vi "TT_Width.vi"(7 "Calibrated Image in":T10(plugin-control), 8 "error in (no error)":errorcluster, 10 "TT side Width Input Cluster":T9 {"Reference ROI Before Transformation"."Contours"."Type" items=["No Selection", "Point", "Line", "Rectangle", "Oval", "Polygon", "Freehand Region", "Annulus", "Unused2", "Unused3", "Broken Line", "Freehand Line", "Rotated Rectangle"]; "Measurement ROI-1 Before transformation"."Contours"."Type" items=["No Selection", "Point", "Line", "Rectangle", "Oval", "Polygon", "Freehand Region", "Annulus", "Unused2", "Unused3", "Broken Line", "Freehand Line", "Rotated Rectangle"]; "Ref Line Edge Options"."Edge Polarity" items=["All Edges", "Rising Edges", "Falling Edges"]; "Ref Line Edge Options"."Minimum Edge Strength" format="%.2f"; "Ref Line Edge Options"."Width" step=2; "Ref Line Edge Options"."Kernel Size" step=2; "Ref Line Options"."Min. Points (%)" min=0.0 max=100.0; "Ref Line Options"."Min. SNR (db)" min=0.0; "Ref Line Options"."Max. Score" min=0.0 max=1024.0; "Ref Line Options"."Min. Score" min=0.0 max=1024.0 step=1.0; "Meas ROI-1 Edge Options"."Edge Polarity" items=["All Edges", "Rising Edges", "Falling Edges"]; "Meas ROI-1 Edge Options"."Minimum Edge Strength" format="%.2f"; "Meas ROI-1 Edge Options"."Width" step=2; "Meas ROI-1 Edge Options"."Kernel Size" step=2}, 11 "Image In":T10) -> (0 "error out":errorcluster, 1 "Measurement 1":sgl, 3 "Angle (Pixel)":dbl, 4 "Array points for Arrow overlay":cluster{"X":sgl, "Y":sgl}[](array[cluster]), 5 "Overlay Arrow Lines":T1)   [LabVIEW 2019, in "Algorithm.lvclass"]
uses:
  FrameworkOverrides/Algorithm.lvclass
  <vilib>/vision/NI_Vision_Development_Module.lvlib
  <vilib>/vision/Measure.llb/Edge Polarity.ctl
  <vilib>/vision/Measure.llb/Edge Options.ctl
  <vilib>/vision/Image Controls.llb/IMAQ Image.ctl
  <vilib>/vision/Measure.llb/Straight Edge Process.ctl
  <vilib>/vision/Measure.llb/Straight Edge Options.ctl
panel:
  out "Second Overlay Line":T2
  out "First Overlay Line":T3
  # "INPUT"
  # "OUTPUT"
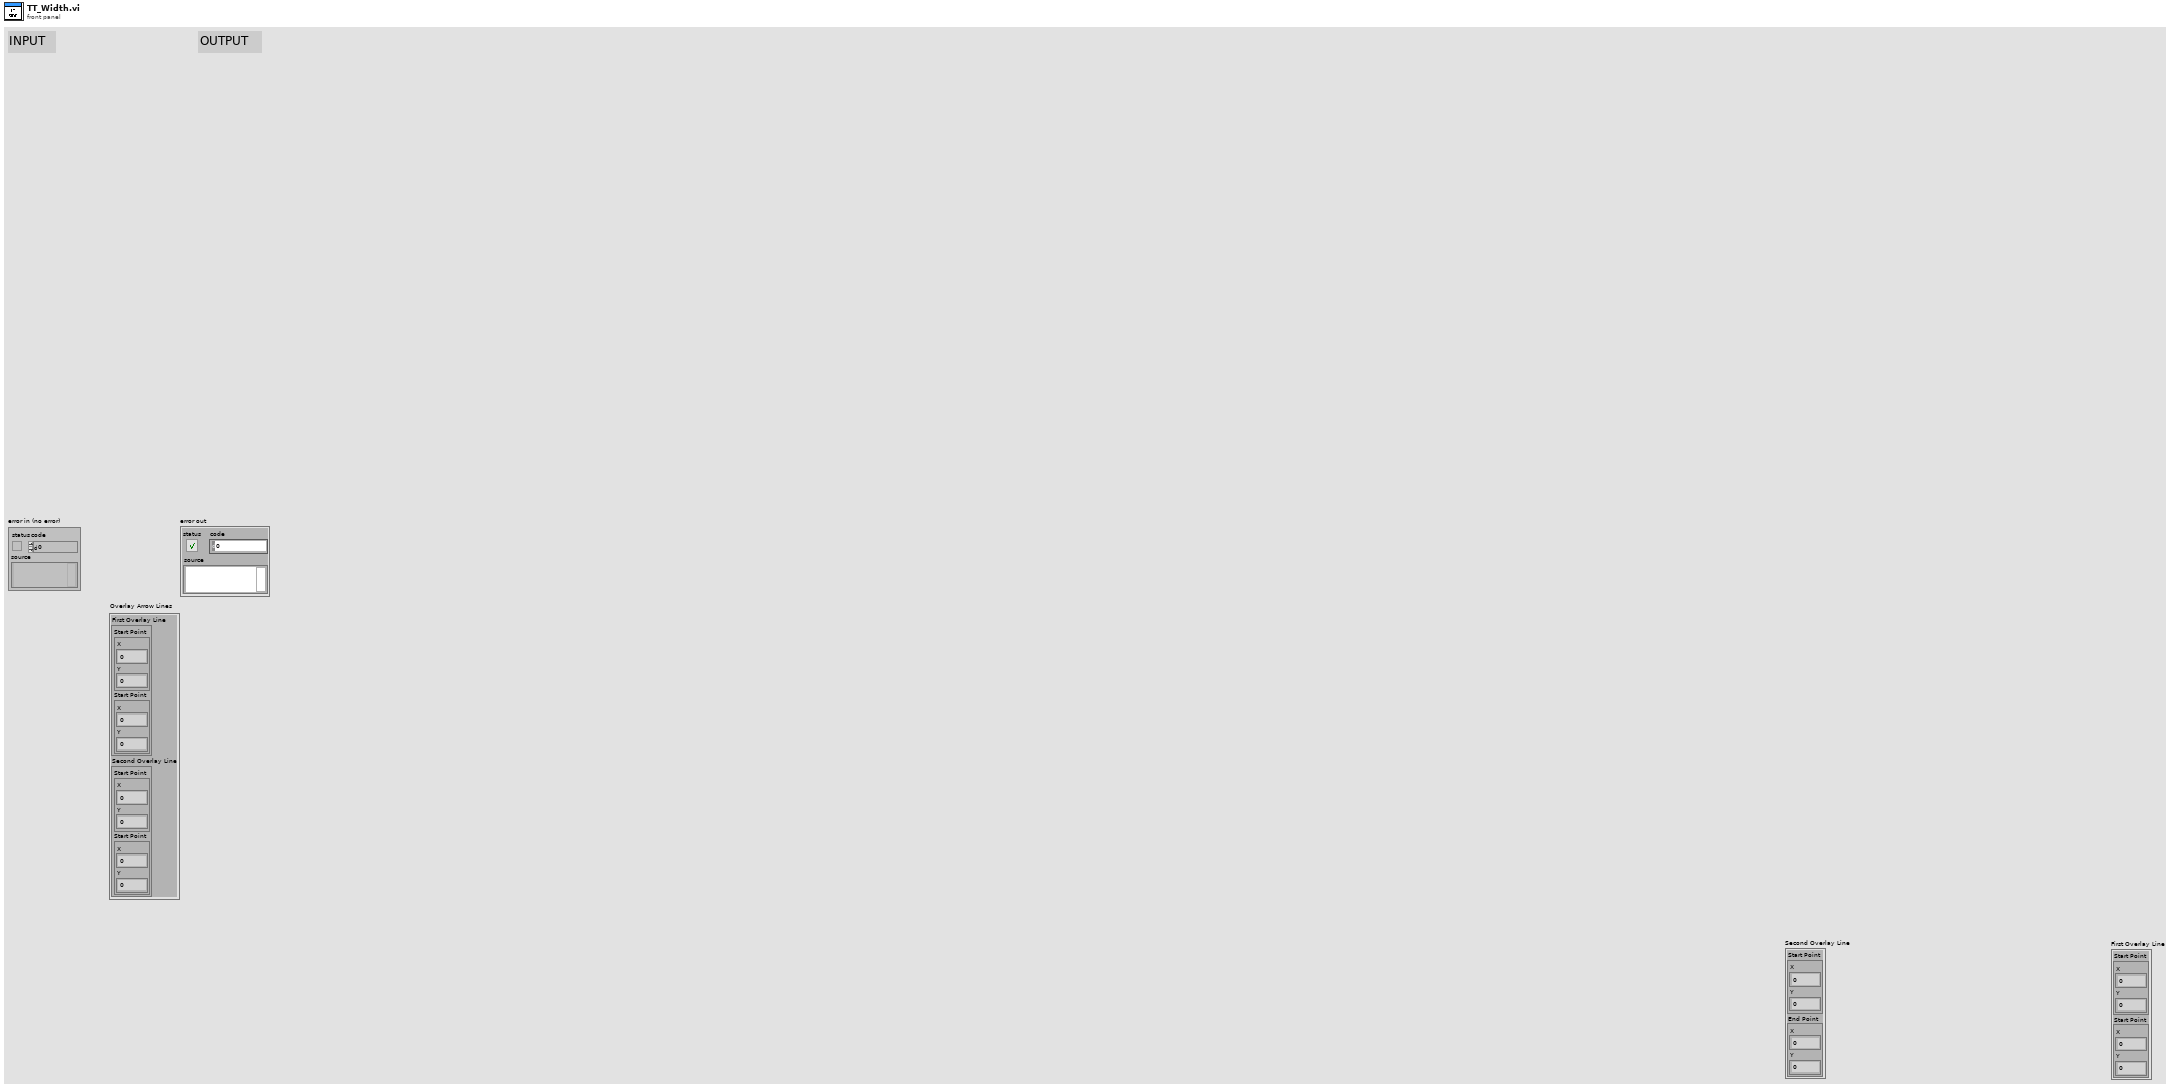
[diagram p1: front panel]
types:
  T1 = cluster{"First Overlay Line ":cluster{"Start Point":cluster{"X":sgl, "Y":sgl}, "Start Point":cluster{"X":sgl, "Y":sgl}}, "Second Overlay Line ":cluster{"Start Point":cluster{"X":sgl, "Y":sgl}, "Start Point":cluster{"X":sgl, "Y":sgl}}}
  T2 = cluster{"Start Point":cluster{"X":sgl, "Y":sgl}, "End Point":cluster{"X":sgl, "Y":sgl}}
  T3 = cluster{"Start Point":cluster{"X":sgl, "Y":sgl}, "Start Point":cluster{"X":sgl, "Y":sgl}}
  T4 = typedef "ROI Descriptor" = cluster{"Global Rectangle":i32[], "Contours":cluster{"ID":enum32{"External", "Internal"}, "Type":u32, "Coordinates":i32[]}[]}
  T5 = typedef "Edge Options.ctl" = cluster{"Edge Polarity":T6, "Kernel Size":u32, "Width":u32, "Minimum Edge Strength":sgl, "Interpolation Type":enum32{"Zero Order", "Bilinear", "Quadratic", "Cubic", "Bilinear Fixed"}, "Data Processing Method":enum32{"Average", "Median"}}
  T6 = typedef "Edge Polarity.ctl" = u32
  T7 = typedef "Straight Edge Options.ctl" = cluster{"Number of Lines":i32, "Type":T8, "Min. Score":dbl, "Max. Score":dbl, "Orientation":dbl, "Angle Range":dbl, "Angle Tolerance":dbl, "Step Size":u32, "Min. SNR (db)":dbl, "Min. Points (%)":dbl, "Hough Iterations":i32}
  T8 = typedef "Straight Edge Process.ctl" = enum32{"First Edge Rake", "Best Edge Rake", "Hough Edge Rake", "First Edge Projection", "Best Edge Projection"}
  T9 = cluster{"AvgMinMax":enum16{"Average", "Max", "Min", "Max2"}, "Center X &Y":cluster{"Center X":dbl, "Center Y":dbl}, "Reference ROI Before Transformation":T4, "Measurement ROI-1 Before transformation":T4, "Ref Line Edge Options":T5, "Ref Line Search Direction":u32, "Ref Line Options":T7, "Meas ROI-1 Edge Options":T5, "Meas ROI-1 Step Size":u32, "Meas ROI-1 Scan Direction":u16, "Meas ROI-1 Process":enum16{"Get First Edge", "Get First + Last Edge", "Get All Edges", "Get Best Edge"}, "OverlayOptions":cluster{"OverlayEnable":bool, "OverlayText":string, "OverlayCoords":i32[], "OverlayAngle":i32, "OverlayTextSize":i32, "OverlayTextColor":string, "OverlayROI":bool, "OverlayRakeLine":bool, "OverlayPoints":bool}}
  T10 = typedef "IMAQ Image.ctl" = refnum<image>
  T11 = cluster{"Left":dbl, "Top":dbl, "Right":dbl, "Bottom":dbl, "Angle":dbl}
  T12 = cluster{"Search Direction":u32, "Edge Options":T5, "Show Search Area":bool, "Show Search Lines":bool, "Show Edges Found":bool, "Show Result":bool, "Search Area Color":u32, "Search Lines Color":u32, "Edge Locations Color":u32, "Result Color":u32, "Overlay Group Name":string}
  T13 = enum16{"Get First Edge", "Get First + Last Edge", "Get All Edges", "Get Best Edge"}
  T14 = cluster{"OverlayEnable":bool, "OverlayText":string, "OverlayCoords":i32[], "OverlayAngle":i32, "OverlayTextSize":i32, "OverlayTextColor":string, "OverlayROI":bool, "OverlayRakeLine":bool, "OverlayPoints":bool}
  T15 = cluster{"ID":enum32{"External", "Internal"}, "Type":u32, "Coordinates":i32[]}[]
  T16 = cluster{"ID":enum32{"External", "Internal"}, "Type":u32, "Coordinates":i32[]}
  T17 = cluster{"Coordinates[0]":i32, "Coordinates[1]":i32, "Coordinates[2]":i32, "Coordinates[3]":i32, "Coordinates[4]":i32}
  T18 = cluster{"Point1 (Pixels)":cluster{"X":sgl, "Y":sgl}, "Point2 (Pixels)":cluster{"X":sgl, "Y":sgl}, "Point1 (Real-World)":cluster{"X":sgl, "Y":sgl}, "Point2 (Real-World)":cluster{"X":sgl, "Y":sgl}, "Angle (Pixel)":dbl, "Angle (Real-World)":dbl, "Score":dbl, "Straightness":dbl, "Average SNR (db)":dbl, "Calibration Valid":bool}[]
  T19 = cluster{"Point1 (Pixels)":cluster{"X":sgl, "Y":sgl}, "Point2 (Pixels)":cluster{"X":sgl, "Y":sgl}, "Point1 (Real-World)":cluster{"X":sgl, "Y":sgl}, "Point2 (Real-World)":cluster{"X":sgl, "Y":sgl}, "Angle (Pixel)":dbl, "Angle (Real-World)":dbl, "Score":dbl, "Straightness":dbl, "Average SNR (db)":dbl, "Calibration Valid":bool}
  T20 = typedef "Edge New.ctl" = cluster{"Location (Pixel)":cluster{"X":sgl, "Y":sgl}, "Location (Real-World)":cluster{"X":sgl, "Y":sgl}, "Distance (Pixel)":dbl, "Distance (Real-World)":dbl, "Strength":dbl, "Noise":dbl, "Rising?":bool}
  T21 = typedef "Search Line.ctl" = cluster{"Start Point":cluster{"X":sgl, "Y":sgl}, "End Point":cluster{"X":sgl, "Y":sgl}, "Edge Info":T20[], "Edge Map":dbl[], "Calibration Valid":bool}
  T22 = cluster{"Start Point":cluster{"X":sgl, "Y":sgl}, "Location (Pixel)":cluster{"X":sgl, "Y":sgl}}
  T23 = cluster{"Location (Pixel)":cluster{"X":sgl, "Y":sgl}, "End Point":cluster{"X":sgl, "Y":sgl}}
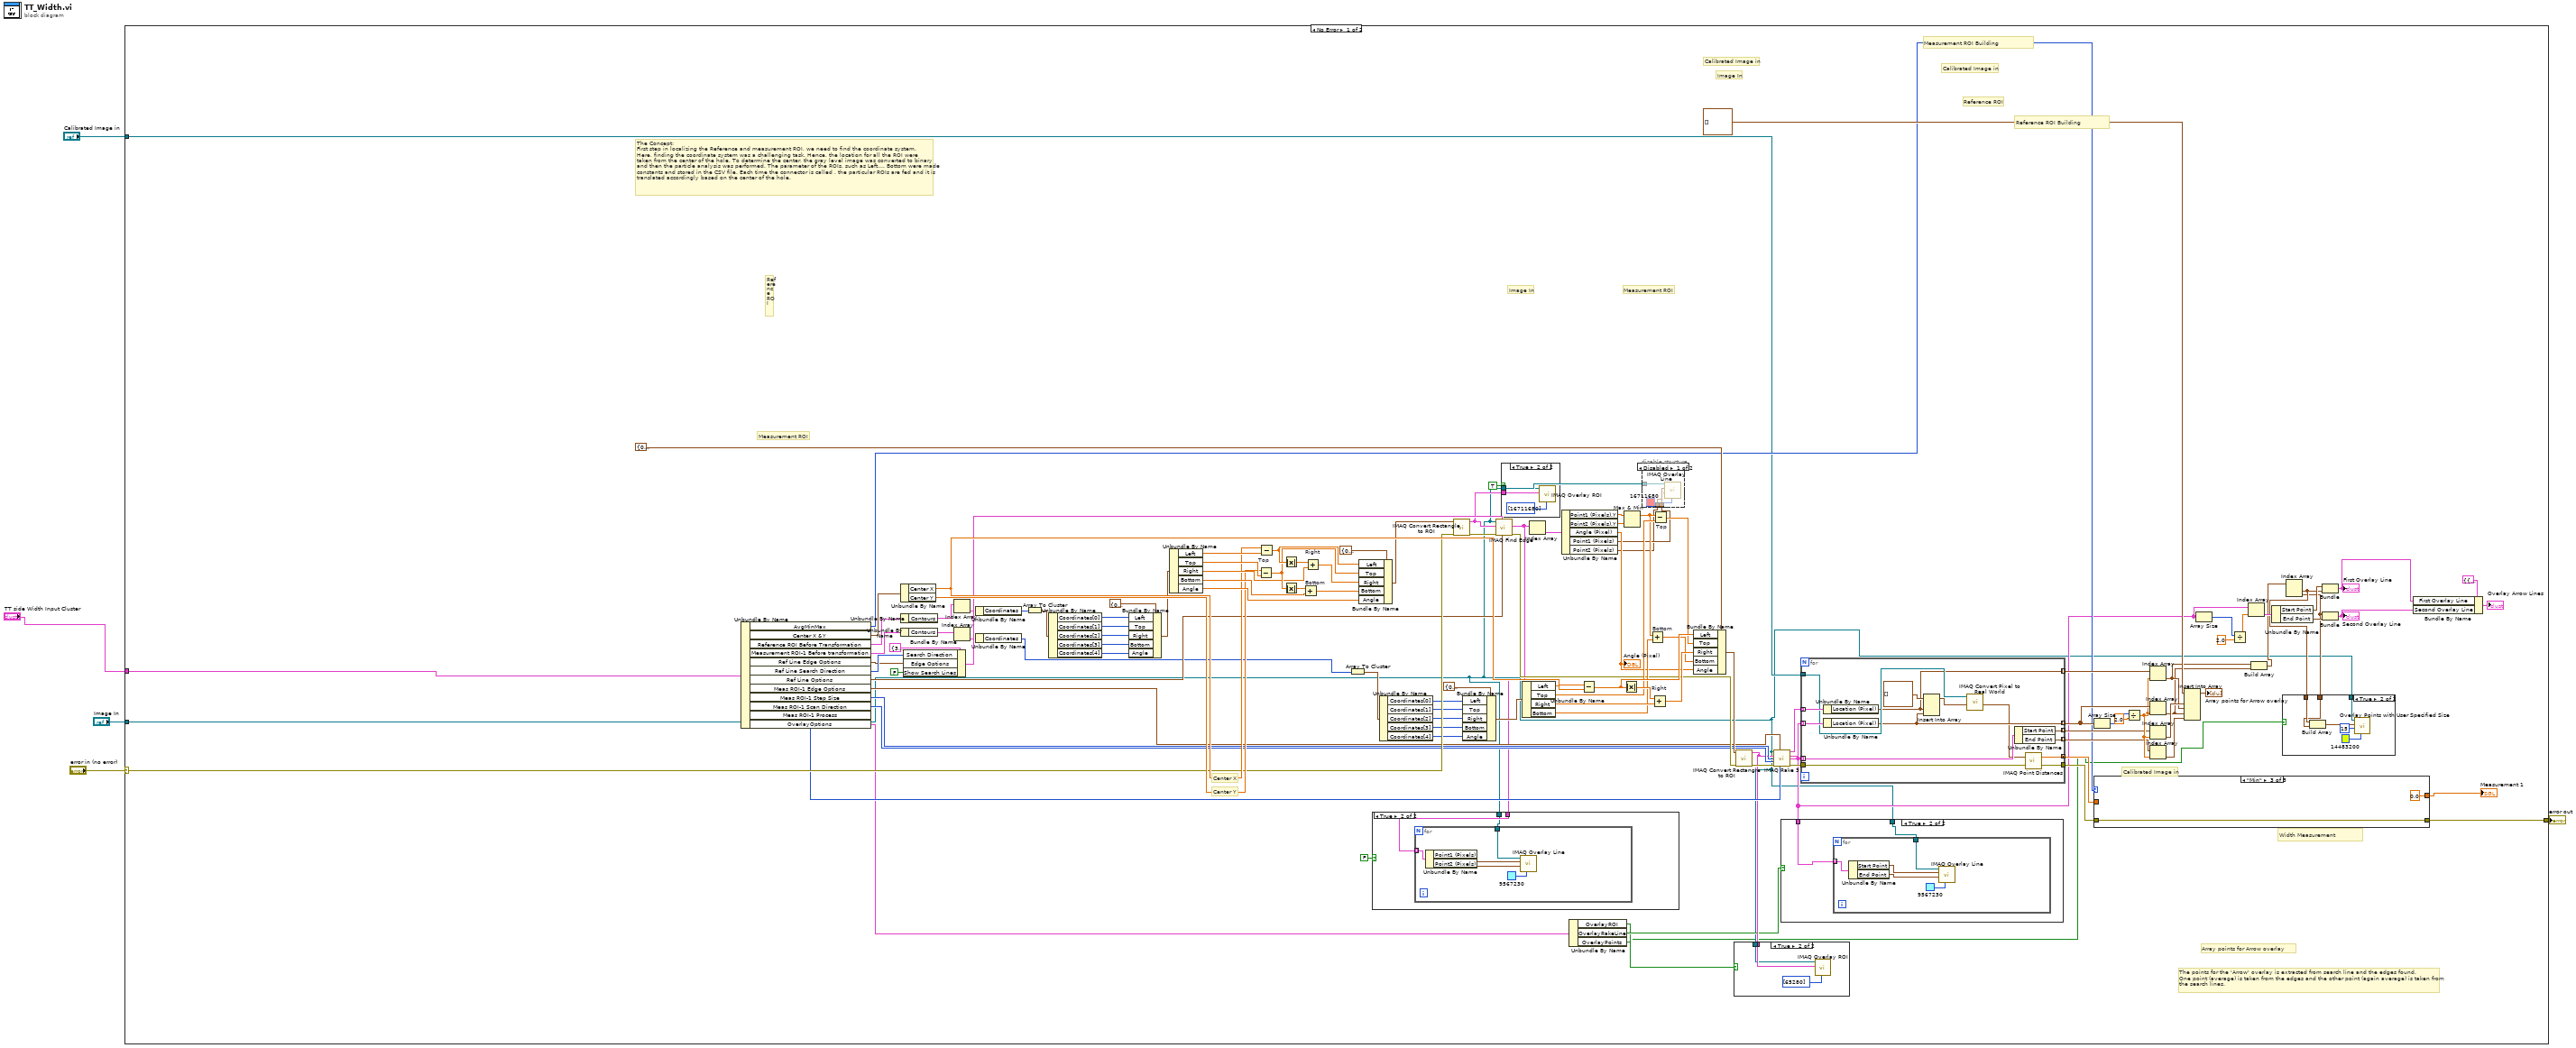
[diagram p0: block diagram]
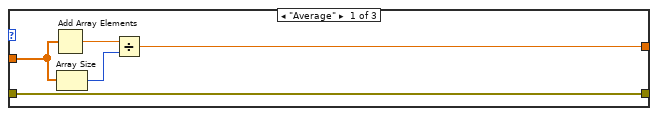
[diagram p8: hidden frame]
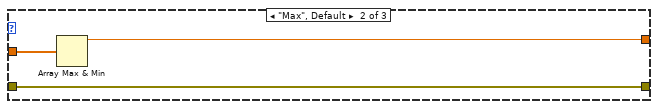
[diagram p9: hidden frame]
diagram:
  n1 = case shown="No Error" "error in (no error)" {
    selector: "error in (no error)" -> [w79 w179]
    tunnel: "Image In" -> [w9 _]
    tunnel: [w91 w179] -> w4
    tunnel: "Calibrated Image in" -> [w37 _]
    tunnel: "TT side Width Input Cluster" -> [w72 _]
    frame No Error {
      # "The points for the 'Arrow' overlay is extracted from search line and the edges found.\nOne point (average) is taken from the edges and the other point (again average) is taken from \nthe search lines."
      # "Array points for Arrow overlay"
      # "The Concept:\nFirst step in localizing the Reference and measurement ROI, we need to find the coordinate system.\nHere, finding the coordinate system was a challenging task. Hence, the location for all the ROI were \ntaken from the center of the hole. To determine the center, the gray level image was converted to binary\nand then the particle analysis was performed. The parameter of the ROIs, such as Left.... Bottom were made \nconstants and stored in the CSV file. Each time the connector is called , the particular ROIs are fed and it is\ntranslated accordingly based on the center of the hole."
      # "Calibrated Image in"
      # "Image In"
      # "Calibrated Image in"
      # "Image In"
      # "Calibrated Image in"
      # "Center Y"
      # "Center X"
      # "Reference ROI"
      # "Measurement ROI"
      # "Width Measurement"
      # "Reference ROI"
      # "Measurement ROI"
      # "Measurement ROI Building"
      # "Reference ROI Building"
      n2 = Unbundle By Name(w72) -> ("AvgMinMax"=w63:enum16{"Average", "Max", "Min", "Max2"}, "Center X &Y"=w62:cluster{"Center X":dbl, "Center Y":dbl}, "Reference ROI Before Transformation"=w56:T4, "Measurement ROI-1 Before transformation"=w46:T4, "Ref Line Edge Options"=w70:T5, "Ref Line Search Direction"=w71:u32, "Ref Line Options"=w68:T7, "Meas ROI-1 Edge Options"=w67:T5, "Meas ROI-1 Step Size"=w66:u32, "Meas ROI-1 Scan Direction"=w65:u16, "Meas ROI-1 Process"=w64:T13, "OverlayOptions"=w28:T14)
      n3 = Unbundle By Name(w62) -> ("Center X"=w81:dbl, "Center Y"=w80:dbl)
      n4 = Unbundle By Name(w56) -> ("Contours"=w55:T15)
      n5 = Unbundle By Name(w46) -> ("Contours"=w59:T15)
      n6 = Bundle By Name(cluster=T12 {"Search Direction"=3, "Edge Options"={"Edge Polarity"=0, "Kernel Size"=3, "Width"=3, "Minimum Edge Strength"=50.0, "Interpolation Type"=enum."Zero Order", "Data Processing Method"=enum."Average"}, "Show Search Area"=FALSE, "Show Search Lines"=FALSE, "Show Edges Found"=FALSE, "Show Result"=FALSE, "Search Area Color"=65280, "Search Lines Color"=255, "Edge Locations Color"=16776960, "Result Color"=16711680, "Overlay Group Name"=""} ("Options"), "Search Direction"=w71, "Edge Options"=w70, "Show Search Lines"=FALSE) -> (w69:T12)
      n7 = Index Array(array=w55) -> (element=w57:T16)  [unwired: 1 in]
      n8 = Index Array(array=w59) -> (element=w60:T16)  [unwired: 1 in]
      n9 = Unbundle By Name(w57) -> ("Coordinates"=w58:i32[])
      n10 = Unbundle By Name(w60) -> ("Coordinates"=w61:i32[])
      n11 = Array To Cluster(array=w58) -> (cluster=w53:T17)
      n12 = Unbundle By Name "Unbundle By Name"(w53) -> ("Coordinates[0]"=w52:i32, "Coordinates[1]"=w51:i32, "Coordinates[2]"=w50:i32, "Coordinates[3]"=w49:i32, "Coordinates[4]"=w48:i32)
      n13 = Bundle By Name(cluster=T11 {"Left"=0.0, "Top"=0.0, "Right"=0.0, "Bottom"=0.0, "Angle"=0.0} ("Measurement ROI-1 Before transformation"), "Left"=w52, "Top"=w51, "Right"=w50, "Bottom"=w49, "Angle"=w48) -> (w47:T11)
      n14 = Unbundle By Name "Unbundle By Name"(w47) -> ("Left"=w107:dbl, "Top"=w106:dbl, "Right"=w105:dbl, "Bottom"=w104:dbl, "Angle"=w103:dbl)
      n15 = Subtract "Top"(x=w80, y=w106) -> (x-y=w114:dbl)
      n16 = Subtract(x=w81, y=w107) -> (x-y=w115:dbl)
      n17 = Absolute Value(x=w115) -> (abs(x)=w118:dbl)
      n18 = Absolute Value(x=w114) -> (abs(x)=w117:dbl)
      n19 = Add "Bottom"(x=w117, y=w104) -> (x+y=w112:dbl)
      n20 = Add "Right"(x=w118, y=w105) -> (x+y=w113:dbl)
      n21 = Array To Cluster(array=w61) -> (cluster=w39:T17)
      n22 = Bundle By Name(cluster=T11 {"Left"=0.0, "Top"=0.0, "Right"=0.0, "Bottom"=0.0, "Angle"=0.0} ("input cluster"), "Left"=w115, "Top"=w114, "Right"=w113, "Bottom"=w112, "Angle"=w103) -> (w36:T11)
      n23 = Unbundle By Name "Unbundle By Name"(w39) -> ("Coordinates[0]"=w41:i32, "Coordinates[1]"=w42:i32, "Coordinates[2]"=w43:i32, "Coordinates[3]"=w44:i32, "Coordinates[4]"=w45:i32)
      n24 = call "IMAQ Convert Rectangle to ROI"("error in (no error)"=w79, "Rectangle"=w36) -> ("error out"=w102:errorcluster, "ROI Descriptor"=w33:T4)  [unwired: 7 in]
      n25 = Bundle By Name(cluster=T11 {"Left"=0.0, "Top"=0.0, "Right"=0.0, "Bottom"=0.0, "Angle"=0.0} ("Measurement ROI-1 Before transformation"), "Left"=w41, "Top"=w42, "Right"=w43, "Bottom"=w44, "Angle"=w45) -> (w38:T11)
      n26 = call "IMAQ Find Edge"("Line Fit Options"=w68, "Options"=w69, "error in (no error)"=w102, "ROI Descriptor"=w33, "Image"=w9) -> ("error out"=w95:errorcluster, "Straight Edges"=w32:T18)  [unwired: 3 in, 2 out]
      n27 = case shown="True" FALSE {
        tunnel: w32 -> [_ w126]
        tunnel: w9 -> [_ w125]
        frame False {
        }
        frame True {
          n28 = for {
            tunnel: w126 -> [w131] mode=indexing
            tunnel: w125 -> [w128]
            n29 = Unbundle By Name(w131) -> ("Point1 (Pixels)"=w130:cluster{"X":sgl, "Y":sgl}, "Point2 (Pixels)"=w129:cluster{"X":sgl, "Y":sgl})
            n30 = call "IMAQ Overlay Line"("Color"=u32 9567230, "End Point"=w129, "Start Point"=w130, "Image"=w128) -> ()  [unwired: 6 in, 2 out]
          }
        }
      }
      n31 = case shown="True" TRUE {
        tunnel: w33 -> [_ w138]
        tunnel: w9 -> [_ w136]
        frame False {
        }
        frame True {
          n32 = call "IMAQ Overlay ROI"("Colors (Green)"=u32[] [16711680], "ROI Descriptor"=w138, "Image"=w136) -> ()  [unwired: 7 in, 2 out]
        }
      }
      n33 = Unbundle By Name(w38) -> ("Left"=w111:dbl, "Top"=w110:dbl, "Right"=w109:dbl, "Bottom"=w108:dbl)
      n34 = Index Array(array=w32) -> (element=w101:T19)  [unwired: 1 in]
      n35 = Unbundle By Name(w101) -> ("Point1 (Pixels).Y"=w78:sgl, "Point2 (Pixels).Y"=w77:sgl, "Angle (Pixel)"=w100:dbl, "Point1 (Pixels)"=w31:cluster{"X":sgl, "Y":sgl}, "Point2 (Pixels)"=w30:cluster{"X":sgl, "Y":sgl})
      "Angle (Pixel)" <- w100
      n36 = Unbundle By Name(w28) -> ("OverlayROI"=w26:bool, "OverlayRakeLine"=w27:bool, "OverlayPoints"=w8:bool)
      n37 = Subtract(x=w81, y=w111) -> (x-y=w122:dbl)
      n38 = Absolute Value(x=w122) -> (abs(x)=w124:dbl)
      n39 = Max & Min(x=w78, y=w77) -> (max(x,y)=w76:sgl)  [unwired: 1 out]
      n40 = disable-structure shown="Disabled" {
        disable-tunnel: w31 -> [w134 _]
        disable-tunnel: w30 -> [w133 _]
        disable-tunnel: w9 -> [w132 _]
        frame Disabled {
          n41 = call "IMAQ Overlay Line"("Color"=u32 16711680, "End Point"=w133, "Start Point"=w134, "Image"=w132) -> ()  [unwired: 6 in, 2 out]
        }
        frame Enabled {
        }
      }
      n42 = Add "Bottom"(x=w76, y=w108) -> (x+y=w119:dbl)
      n43 = Add "Right"(x=w124, y=w109) -> (x+y=w120:dbl)
      n44 = Subtract "Top"(x=w76, y=w110) -> (x-y=w121:dbl)
      n45 = Bundle By Name(cluster=T11 {"Left"=0.0, "Top"=0.0, "Right"=0.0, "Bottom"=0.0, "Angle"=0.0} ("input cluster"), "Left"=w122, "Top"=w121, "Right"=w120, "Bottom"=w119, "Angle"=w100) -> (w96:T11)
      n46 = call "IMAQ Convert Rectangle to ROI"("error in (no error)"=w95, "Rectangle"=w96) -> ("error out"=w94:errorcluster, "ROI Descriptor"=w34:T4)  [unwired: 7 in]
      n47 = case shown="True" w26 {
        tunnel: w34 -> [_ w147]
        tunnel: w9 -> [_ w145]
        frame False {
        }
        frame True {
          n48 = call "IMAQ Overlay ROI"("Colors (Green)"=u32[] [65280], "ROI Descriptor"=w147, "Image"=w145) -> ()  [unwired: 7 in, 2 out]
        }
      }
      n49 = call "IMAQ Rake 3"("Image"=w9, "Edge Options"=w67, "ROI Descriptor"=w34, "Step Size"=w66, "Scan Direction"=w65, "error in (no error)"=w94, "Process"=w64) -> ("First Edges"=w98:T20[], "Last Edges"=w99:T20[], "Search Lines"=w13:T21[], "error out"=w93:errorcluster)  [unwired: 5 in]
      n50 = case shown="True" w27 {
        tunnel: w13 -> [_ w149]
        tunnel: w9 -> [_ w148]
        frame False {
        }
        frame True {
          n51 = for {
            tunnel: w149 -> [w154] mode=indexing
            tunnel: w148 -> [w151]
            n52 = Unbundle By Name(w154) -> ("Start Point"=w153:cluster{"X":sgl, "Y":sgl}, "End Point"=w152:cluster{"X":sgl, "Y":sgl})
            n53 = call "IMAQ Overlay Line"("Color"=u32 9567230, "End Point"=w152, "Start Point"=w153, "Image"=w151) -> ()  [unwired: 6 in, 2 out]
          }
        }
      }
      n54 = for {
        tunnel: w98 -> [w178] mode=indexing
        tunnel: w99 -> [w177] mode=indexing
        tunnel: [w175] -> w97 mode=concatenating
        tunnel: w93 -> [w174]
        tunnel: [w173] -> w92
        tunnel: w37 -> [w168]
        tunnel: w13 -> [w171] mode=indexing
        tunnel: [w167] -> w88 mode=indexing
        tunnel: [w165] -> w87 mode=indexing
        tunnel: [w170] -> w85 mode=indexing
        tunnel: [w169] -> w84 mode=indexing
        n55 = Unbundle By Name(w178) -> ("Location (Pixel)"=w165:cluster{"X":sgl, "Y":sgl})
        n56 = Unbundle By Name(w177) -> ("Location (Pixel)"=w167:cluster{"X":sgl, "Y":sgl})
        n57 = Insert Into Array(array=cluster{"X":sgl, "Y":sgl}[] [], new element #1=w165, new element #2=w167) -> (w172:cluster{"X":sgl, "Y":sgl}[])  [unwired: 1 in]
        n58 = call "IMAQ Convert Pixel to Real World"("Array of Pixel Coordinates"=w172, "Calibrated Image"=w168) -> ("Array of Real World Coordinates"=w166:cluster{"X":sgl, "Y":sgl}[])  [unwired: 4 in, 5 out]
        n59 = Unbundle By Name(w171) -> ("Start Point"=w170:cluster{"X":sgl, "Y":sgl}, "End Point"=w169:cluster{"X":sgl, "Y":sgl})
        n60 = call "IMAQ Point Distances"("Points"=w166, "error in (no error)"=w174) -> ("Distances"=w175:sgl[], "error out"=w173:errorcluster)  [unwired: 3 in]
      }
      n61 = Array Size(array=w88) -> (size(s)=w89:i32)
      n62 = case shown="\"Min\"" w63 {
        tunnel: w97 -> [w159 w161 _]
        tunnel: w92 -> [w156 w162 w164]
        tunnel: [w156 w162 w164] -> w91
        tunnel: [w155 w160 sgl 0.0] -> w35
        frame "Average" {
          n63 = Add Array Elements(numeric array=w159) -> (sum=w158:sgl)
          n64 = Array Size(array=w159) -> (size(s)=w157:i32)
          n65 = Divide(x=w158, y=w157) -> (x/y=w155:sgl)
        }
        frame "Max", Default {
          n66 = Array Max & Min(array=w161) -> (max value=w160:sgl)  [unwired: 3 out]
        }
        frame "Min" {
        }
      }
      "Measurement 1" <- w35
      n67 = Divide(x=w89, y=2.0) -> (x/y=w86:dbl)
      n68 = Index Array(array=w87, index=w86) -> (element=w16:cluster{"X":sgl, "Y":sgl})
      n69 = Index Array(array=w88, index=w86) -> (element=w15:cluster{"X":sgl, "Y":sgl})
      n70 = Index Array(array=w85, index=w86) -> (element=w74:cluster{"X":sgl, "Y":sgl})
      n71 = Index Array(array=w84, index=w86) -> (element=w82:cluster{"X":sgl, "Y":sgl})
      n72 = Insert Into Array(array=cluster{"X":sgl, "Y":sgl}[] [], new element #1=w74, new element #2=w16, new element #3=w15, new element #4=w82) -> (→"Array points for Arrow overlay":cluster{"X":sgl, "Y":sgl}[])  [unwired: 1 in]
      n73 = Array Size(array=w13) -> (size(s)=w18:i32)
      n74 = Divide(x=w18, y=2.0) -> (x/y=w17:dbl)
      n75 = Index Array(array=w13, index=w17) -> (element=w25:T21)
      n76 = Build Array(w16, w15) -> (w14:cluster{"X":sgl, "Y":sgl}[])
      n77 = Unbundle By Name(w25) -> ("Start Point"=w24:cluster{"X":sgl, "Y":sgl}, "End Point"=w23:cluster{"X":sgl, "Y":sgl})
      n78 = Index Array(array=w14) -> (element #1=w11:cluster{"X":sgl, "Y":sgl}, element #2=w10:cluster{"X":sgl, "Y":sgl})  [unwired: 2 in]
      n79 = case shown="True" w8 {
        tunnel: w11 -> [_ w144]
        tunnel: w10 -> [_ w143]
        tunnel: w9 -> [_ w141]
        frame False {
        }
        frame True {
          n80 = Build Array(w144, w143) -> (w142:cluster{"X":sgl, "Y":sgl}[])
          n81 = call "Overlay Points with User Specified Size.vi"("Color"=u32 14483200, "Point Diameter (5)"=u32 15, "Points"=w142, "Image In"=w141) -> ()  [unwired: 6 in, 2 out]
        }
      }
      n82 = Bundle("Start Point"=w24, "Location (Pixel)"=w11) -> (w21:T22)  [unwired: 1 in]
      "First Overlay Line" <- w21
      n83 = Bundle("Location (Pixel)"=w10, "End Point"=w23) -> (w20:T23)  [unwired: 1 in]
      "Second Overlay Line" <- w20
      n84 = Bundle By Name(cluster=T1 {"First Overlay Line "={"Start Point"={"X"=0.0, "Y"=0.0}, "Start Point"={"X"=0.0, "Y"=0.0}}, "Second Overlay Line "={"Start Point"={"X"=0.0, "Y"=0.0}, "Start Point"={"X"=0.0, "Y"=0.0}}}, "First Overlay Line"=w21, "Second Overlay Line"=w20) -> (→"Overlay Arrow Lines":T1)
    }
    frame Error {
    }
  }
  "error out" <- w4
